vi "R_tau.vi"(9 "fphi":dbl, 10 "Constants and System Parameters":T1) -> (2 "R_tau":dbl)   [LabVIEW 2018]
uses:
  Constants and System Parameters.ctl
panel:
  out "eta":dbl
  out "R2":dbl
  out "R1":dbl
  out "cos(x)":dbl
  out "d":dbl
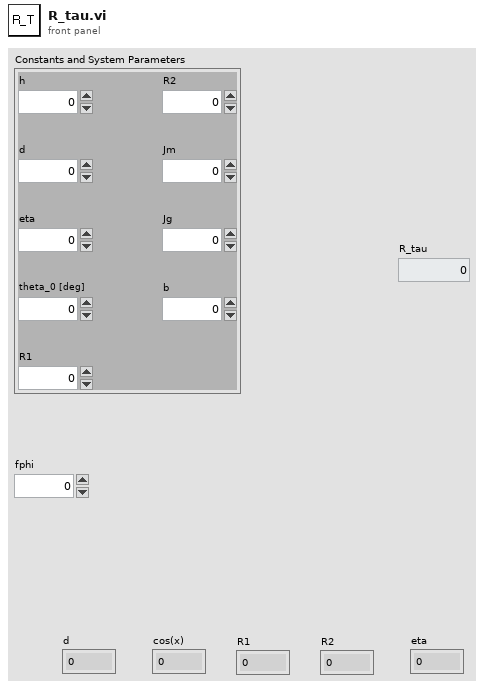
[diagram p1: front panel]
types:
  T1 = typedef "Constants and System Parameters.ctl" = cluster{"h":dbl, "d":dbl, "eta":dbl, "theta_0 [deg]":dbl, "R1":dbl, "R2":dbl, "Jm":dbl, "Jg":dbl, "b":dbl}
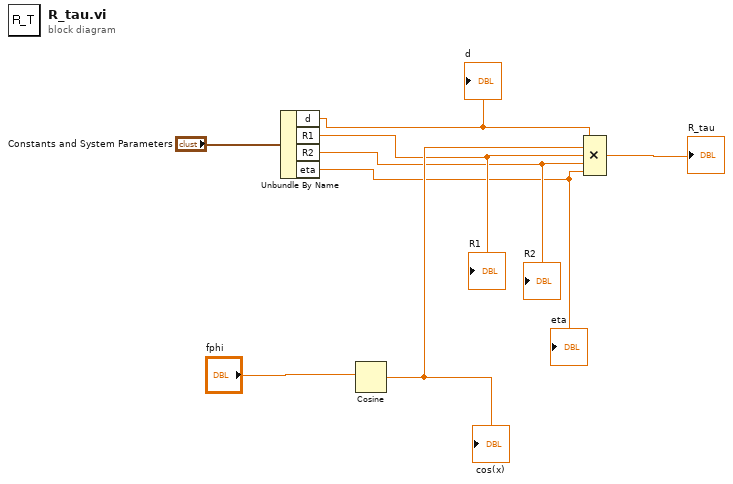
[diagram p0: block diagram]
diagram:
  n1 = Unbundle By Name("Constants and System Parameters") -> ("d"=w4:dbl, "R1"=w3:dbl, "R2"=w2:dbl, "eta"=w1:dbl)
  "d" <- w4
  "R1" <- w3
  "R2" <- w2
  "eta" <- w1
  n2 = Cosine(x="fphi") -> (cos(x)=w8:dbl)
  "cos(x)" <- w8
  n3 = Compound Arithmetic op=MULTIPLY(w4, w8, w3, w2, w1) -> (→"R_tau":dbl)
